vi "accept.vi"(8 "error in":errorcluster, 10 "connection ID":refnum<k5>, 11 "TLS HTTP handler dataset in":refnum<class "TLS HTTP handler dataset.lvclass">) -> (0 "error out":errorcluster, 2 "lvlibretls connection":refnum<class "lvlibretls connection.lvclass">)   [LabVIEW 2016, in "TLS HTTP handler dataset.lvclass"]
uses:
  TLS HTTP handler dataset.lvclass
  lvlibtls/socket connection/lvlibretls connection.lvclass
  TLS HTTP handler dataset.lvclass/TLS HTTP handler dataset.ctl
  lvlibtls/server/lvlibretls server listener.lvclass
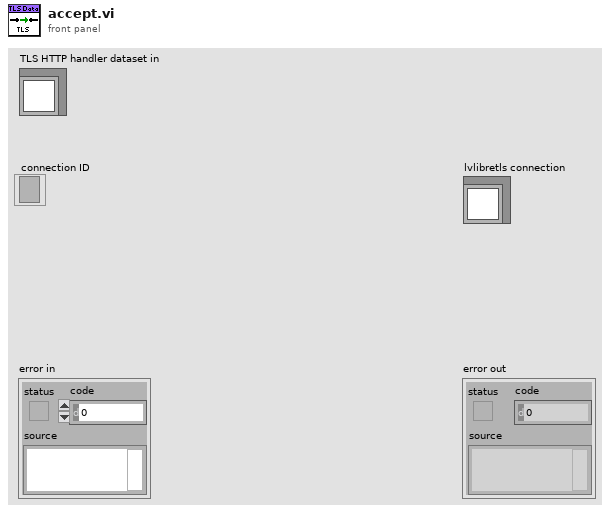
[diagram p1: front panel]
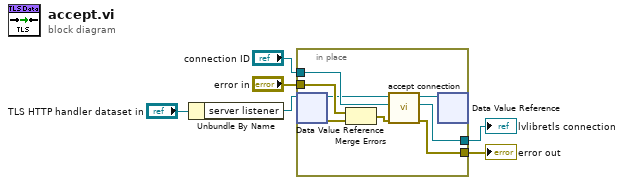
[diagram p0: block diagram]
diagram:
  n1 = Unbundle By Name("TLS HTTP handler dataset in") -> ("server listener"=w1:refnum<data-value>)
  n2 = in-place {
    in-place-border: [w14] -> w5
    in-place-border: [w13] -> w4
    in-place-border: "error in" -> [w12]
    in-place-border: "connection ID" -> [w11]
    n3 = in-place-dvr #1(w1) -> (w10:refnum<class "lvlibretls server listener.lvclass">, w7:errorcluster)
    n4 = Merge Errors(w12, w7) -> (w8:errorcluster)
    n5 = call "accept connection.vi"("error in"=w8, "connection ID"=w11, "lvlibretls server listener in"=w10) -> ("error out"=w13:errorcluster, "lvlibretls connection"=w14:refnum<class "lvlibretls connection.lvclass">, "lvlibretls server listener out"=w9:refnum<class "lvlibretls server listener.lvclass">)  [unwired: 6 in]
    n6 = in-place-dvr #1(w9) -> ()  [unwired: 2 out]
  }
  "error out" <- w4
  "lvlibretls connection" <- w5
